vi "FourFlippingCoin.vi"() -> ()   [LabVIEW 2017]
uses:
  <vilib>/Analysis/NI_AALBase.lvlib
panel:
  out "Waveform Graph":i32[](graph)
  out "Array 2":i16[](array[numeric])
  out "X Values":dbl[](array[numeric]) format="%0.2f"
  out "Histogram: h(x)":i32[](array[numeric])
  in  "The total  number fo Trails":i32=8
  out "Heads":i16
  out "0, 1":i16[](array[numeric])
  out "Array":bool[](array[boolean])
  out "Coin 4":bool
  out "Coin 3":bool
  out "Coin 2":bool
  out "Coin 1":bool
  # "Heads = Lit"
  # "Tails = Unlit"
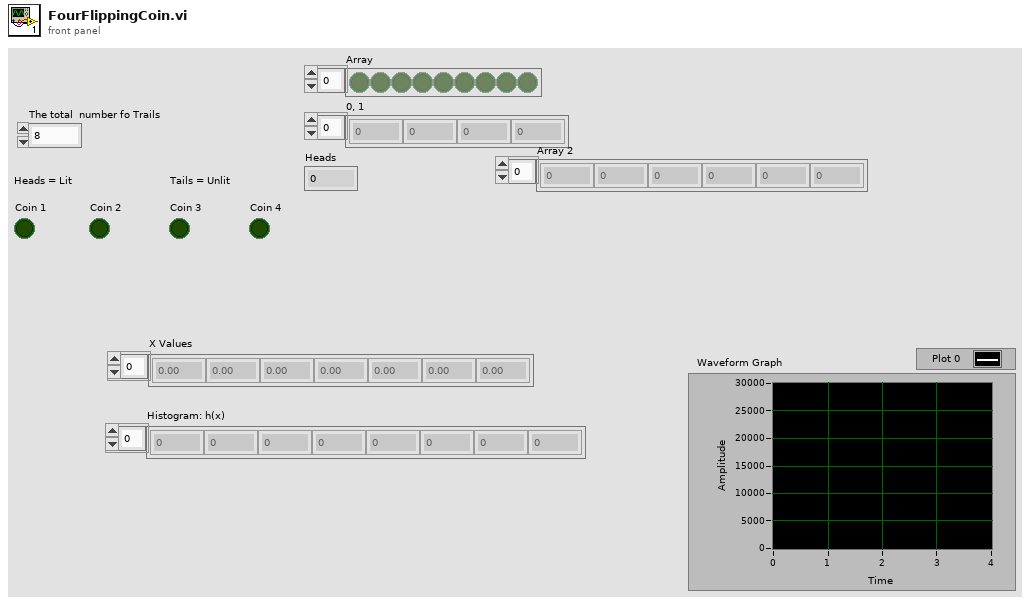
[diagram p1: front panel]
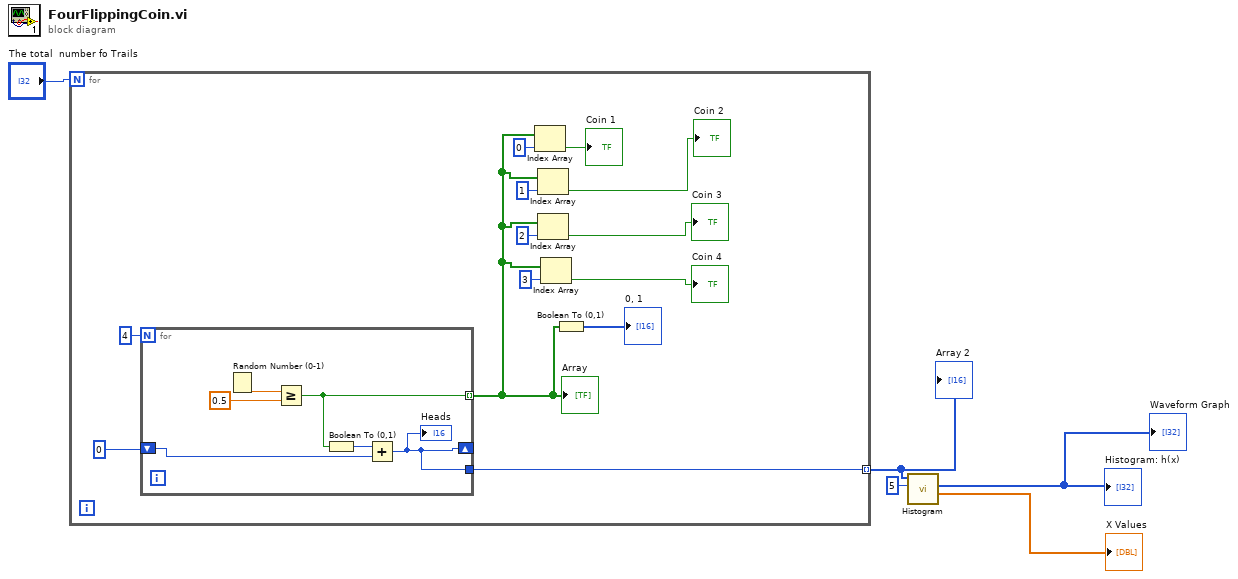
[diagram p0: block diagram]
diagram:
  n1 = for {
    N: "The total  number fo Trails" -> [_]
    tunnel: [w6] -> w3 mode=indexing
    n2 = for {
      N: 4 -> [_]
      tunnel: [w22] -> w15 mode=indexing
      shift-right: [w19] -> _
      shift-left: i16 0 ("y") -> [w20]
      tunnel: [w19] -> w6
      n3 = Random Number (0-1)() -> (number: 0 to 1=w23:dbl)
      n4 = Greater Or Equal?(x=w23, y=0.5) -> (x >= y?=w22:bool)
      n5 = Boolean To (0,1)(Boolean=w22) -> (0, 1=w21:i16)
      n6 = Add(x=w21, y=w20) -> (x+y=w19:i16)
      "Heads" <- w19
    }
    "Array" <- w15
    n7 = Index Array(array=w15, index=0) -> (element=→"Coin 1":bool)
    n8 = Index Array(array=w15, index=1) -> (element=→"Coin 2":bool)
    n9 = Index Array(array=w15, index=2) -> (element=→"Coin 3":bool)
    n10 = Index Array(array=w15, index=3) -> (element=→"Coin 4":bool)
    n11 = Boolean To (0,1)(Boolean=w15) -> (0, 1=→"0, 1":i16[])
  }
  "Array 2" <- w3
  n12 = call <vilib>:"Histogram.vi"("intervals"=5, "X"=w3) -> ("X Values"=→"X Values":dbl[], "Histogram: h(x)"=→"Histogram: h(x)" →"Waveform Graph":i32[])  [unwired: 6 in, 2 out]
